vi "扫描脚本.vi"(4 "4-wire":bool, 6 "扫描":T1 {"测试参数"."反向极限电流(mA)" min=0.0 max=3000.0; "测试参数"."反向电压(V)" min=0.0 max=40.0; "测试参数"."正向极限电流(mA)" min=0.0 max=3000.0; "测试参数"."正向电压(V)" min=0.0 max=40.0; "时序参数"."反改变量(V)" min=0.0 max=40.0 step=5e-06; "时序参数"."正改变量(V)" min=0.0 max=40.0 step=5e-06; "时序参数"."nplc" min=0.001}, 8 "错误输入（无错误）":errorcluster, 11 "方向(T:正向)":bool=TRUE) -> (0 "错误输出":errorcluster, 1 "Script":string)   [LabVIEW 2021]
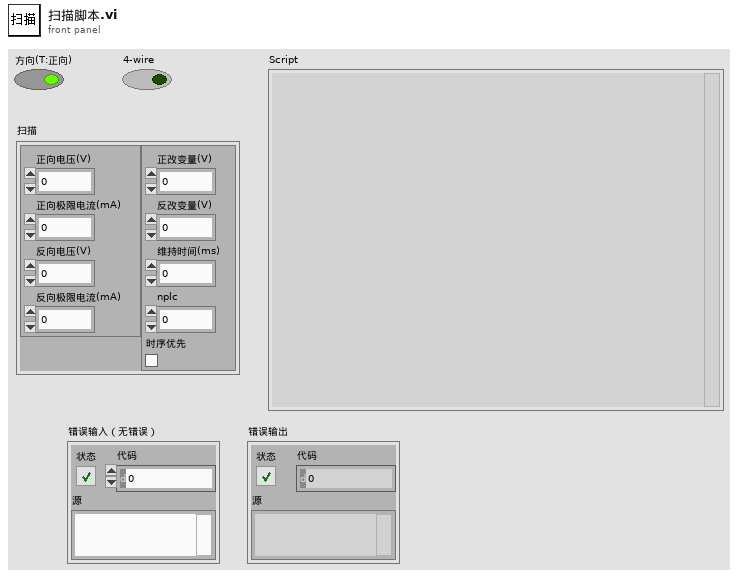
[diagram p1: front panel]
types:
  T1 = typedef "扫描参数.ctl" = cluster{"测试参数":cluster{"正向电压(V)":dbl, "正向极限电流(mA)":dbl, "反向电压(V)":dbl, "反向极限电流(mA)":dbl}, "时序参数":cluster{"正改变量(V)":dbl, "反改变量(V)":dbl, "维持时间(ms)":dbl, "nplc":dbl, "时序优先":bool}}
  T2 = cluster{"正改变量(V)":dbl, "反改变量(V)":dbl, "维持时间(ms)":dbl, "nplc":dbl, "时序优先":bool}
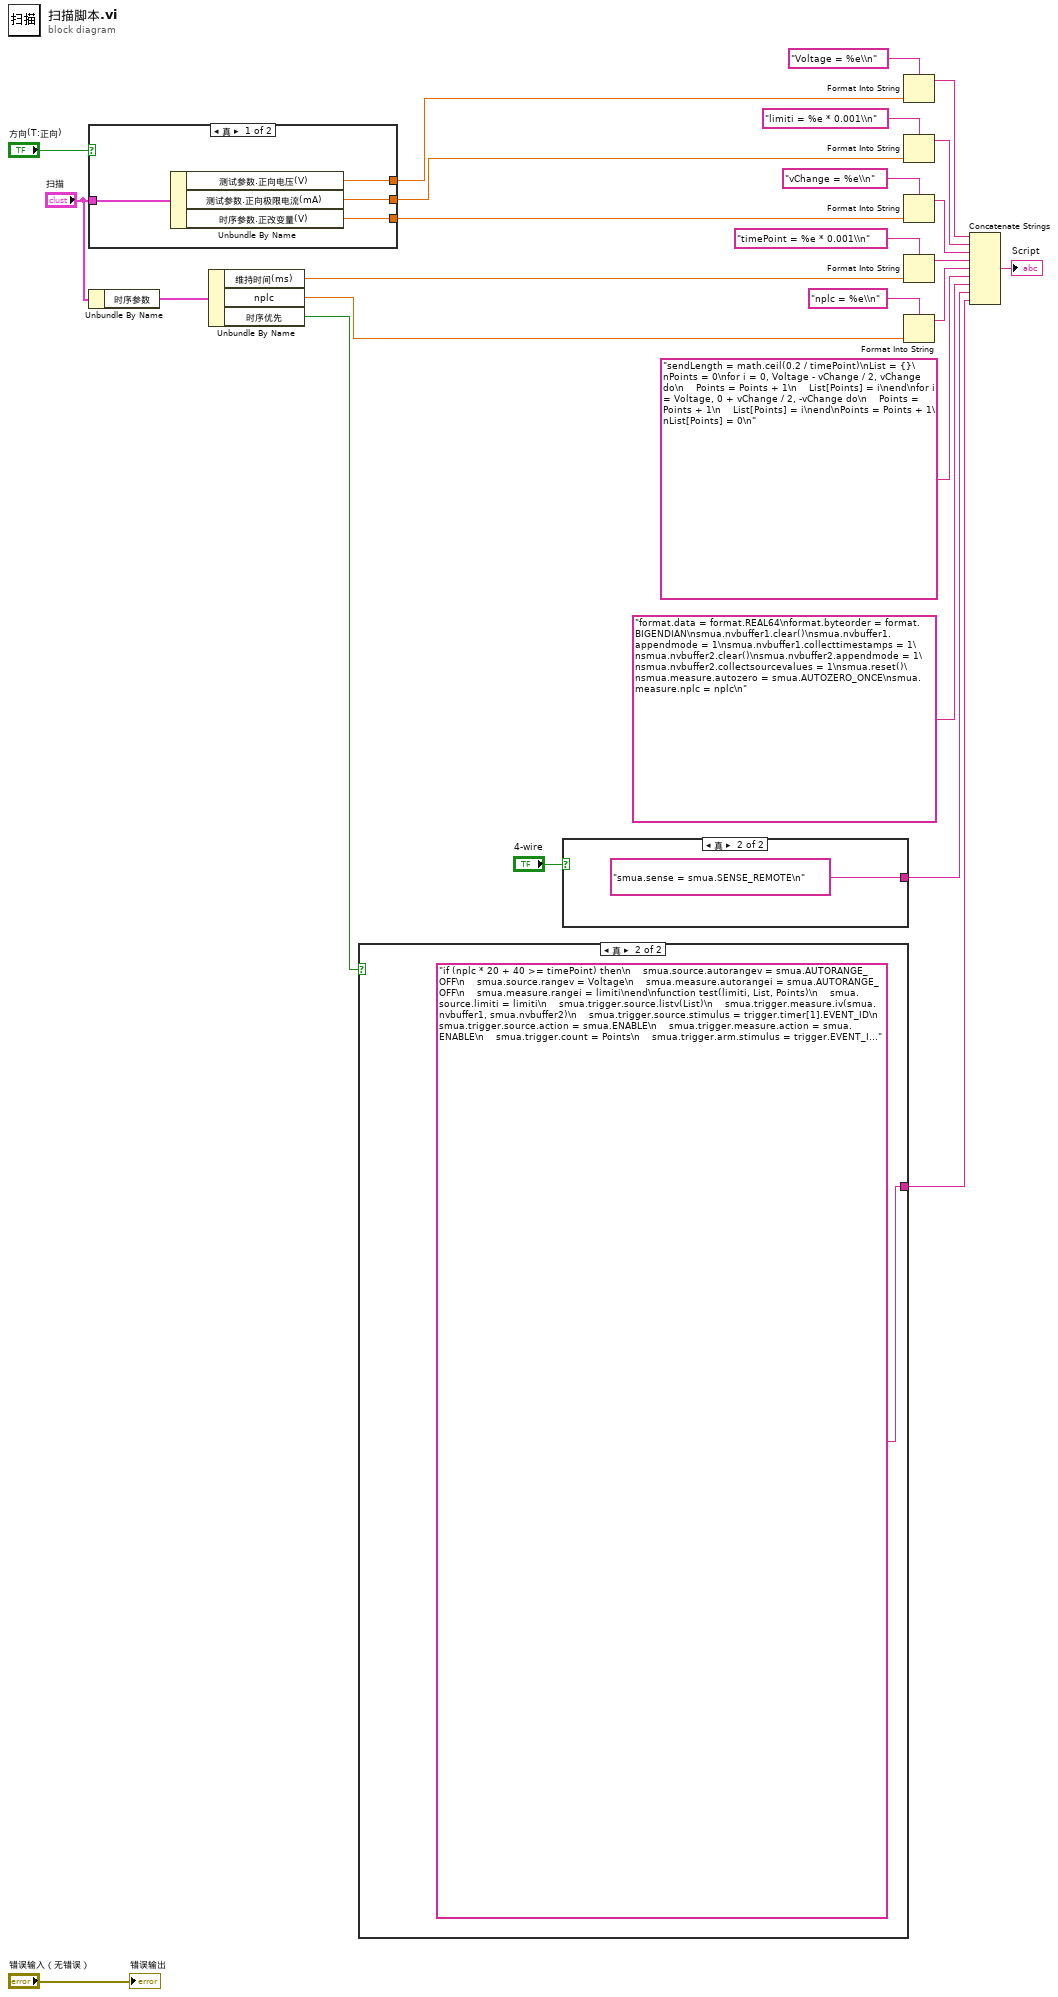
[diagram p0: block diagram]
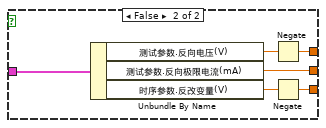
[diagram p2: hidden frame]
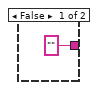
[diagram p3: hidden frame]
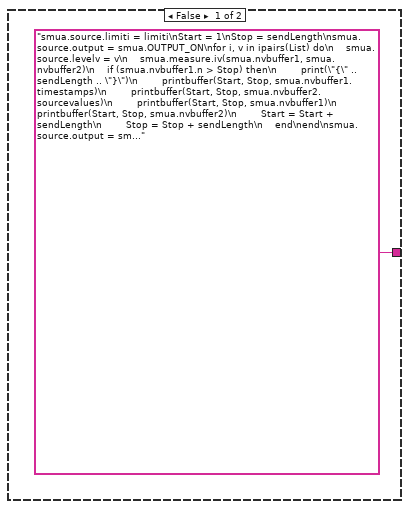
[diagram p4: hidden frame]
diagram:
  n1 = case shown="真" "方向(T:正向)" {
    tunnel: [w30 w35] -> w12
    tunnel: [w29 w32] -> w9
    tunnel: [w28 w33] -> w3
    tunnel: "扫描" -> [w27 w31]
    frame True {
      n2 = Unbundle By Name(w27) -> ("测试参数.正向电压(V)"=w30:dbl, "测试参数.正向极限电流(mA)"=w29:dbl, "时序参数.正改变量(V)"=w28:dbl)
    }
    frame False {
      n3 = Unbundle By Name(w31) -> ("测试参数.反向电压(V)"=w36:dbl, "测试参数.反向极限电流(mA)"=w32:dbl, "时序参数.反改变量(V)"=w34:dbl)
      n4 = Negate(x=w36) -> (-x=w35:dbl)
      n5 = Negate(x=w34) -> (-x=w33:dbl)
    }
  }
  n6 = Unbundle By Name("扫描") -> ("时序参数"=w15:T2)
  n7 = Unbundle By Name(w15) -> ("维持时间(ms)"=w5:dbl, "nplc"=w8:dbl, "时序优先"=w4:bool)
  n8 = case shown="真" w4 {
    tunnel: ["smua.source.limiti = limiti\nStart = 1\nStop = sendLength\nsmua.source.output = smua.OUTPUT_ON\nfor i, v in ipairs(List) do\n    smua.source.levelv = v\n    smua.measure.iv(smua.nvbuffer1, smua.nvbuffer2)\n    if (smua.nvbuffer1.n > Stop) then\n        print(\"{\" .. sendLength .. \"}\")\n        printbuffer(Start, Stop, smua.nvbuffer1.timestamps)\n        printbuffer(Start, Stop, smua.nvbuffer2.sourcevalues)\n        printbuffer(Start, Stop, smua.nvbuffer1)\n        printbuffer(Start, Stop, smua.nvbuffer2)\n        Start = Start + sendLength\n        Stop = Stop + sendLength\n    end\nend\nsmua.source.output = smua.OUTPUT_OFF\nStop = Points\nprint(\"{\" .. Stop - Start + 1 .. \"}\")\nprintbuffer(Start, Stop, smua.nvbuffer1.timestamps)\nprintbuffer(Start, Stop, smua.nvbuffer2.sourcevalues)\nprintbuffer(Start, Stop, smua.nvbuffer1)\nprintbuffer(Start, Stop, smua.nvbuffer2)\nprint(\"{done}\")\nreset()" "if (nplc * 20 + 40 >= timePoint) then\n    smua.source.autorangev = smua.AUTORANGE_OFF\n    smua.source.rangev = Voltage\n    smua.measure.autorangei = smua.AUTORANGE_OFF\n    smua.measure.rangei = limiti\nend\nfunction test(limiti, List, Points)\n    smua.source.limiti = limiti\n    smua.trigger.source.listv(List)\n    smua.trigger.measure.iv(smua.nvbuffer1, smua.nvbuffer2)\n    smua.trigger.source.stimulus = trigger.timer[1].EVENT_ID\n    smua.trigger.source.action = smua.ENABLE\n    smua.trigger.measure.action = smua.ENABLE\n    smua.trigger.count = Points\n    smua.trigger.arm.stimulus = trigger.EVENT_ID\n    trigger.timer[1].reset()\n    trigger.timer[1].stimulus = smua.trigger.ARMED_EVENT_ID\n    trigger.timer[1].passthrough = false\n    trigger.timer[1].delay = timePoint\n    trigger.timer[1].count = Points\n    smua.trigger.initiate()\n    smua.trigger.arm.set()\nend\nfunction sendData()\n    repeat\n        if (bit.test(status.operation.instrument.smua.condition, 4) == false) then\n            return\n        elseif (smua.nvbuffer1.n > Stop) then\n            print(\"{\" .. sendLength .. \"}\")\n            printbuffer(Start, Stop, smua.nvbuffer1.timestamps)\n            printbuffer(Start, Stop, smua.nvbuffer2.sourcevalues)\n            printbuffer(Start, Stop, smua.nvbuffer1)\n            printbuffer(Start, Stop, smua.nvbuffer2)\n            Start = Start + sendLength\n            Stop = Stop + sendLength\n        end\n        delay(timePoint)\n    until (false)\nend\nfunction sendLastData()\n    Stop = smua.nvbuffer1.n\n    print(\"{\" .. Stop - Start + 1 .. \"}\")\n    printbuffer(Start, Stop, smua.nvbuffer1.timestamps)\n    printbuffer(Start, Stop, smua.nvbuffer2.sourcevalues)\n    printbuffer(Start, Stop, smua.nvbuffer1)\n    printbuffer(Start, Stop, smua.nvbuffer2)\n    print(\"{done}\")\nend\nStart = 1\nStop = sendLength\nsmua.source.output = smua.OUTPUT_ON\ntest(limiti, List, Points)\nsendData()\nsmua.source.output = smua.OUTPUT_OFF\nsendLastData()\nreset()"] -> w18
    frame False {
    }
    frame True {
    }
  }
  n9 = case shown="真" "4-wire" {
    tunnel: ["" "smua.sense = smua.SENSE_REMOTE\n"] -> w17
    frame False {
    }
    frame True {
    }
  }
  n10 = Format Into String(format string="Voltage = %e\\n" ("格式字符串"), w12) -> (resulting string=w23:string)  [unwired: 2 in, 1 out]
  n11 = Format Into String(format string="limiti = %e * 0.001\\n" ("格式字符串"), w9) -> (resulting string=w10:string)  [unwired: 2 in, 1 out]
  n12 = Format Into String(format string="vChange = %e\\n" ("格式字符串"), w3) -> (resulting string=w11:string)  [unwired: 2 in, 1 out]
  n13 = Format Into String(format string="timePoint = %e * 0.001\\n", w5) -> (resulting string=w7:string)  [unwired: 2 in, 1 out]
  n14 = Format Into String(format string="nplc = %e\\n", w8) -> (resulting string=w6:string)  [unwired: 2 in, 1 out]
  n15 = Concatenate Strings(w23, w10, w11, w7, w6, "sendLength = math.ceil(0.2 / timePoint)\nList = {}\nPoints = 0\nfor i = 0, Voltage - vChange / 2, vChange do\n    Points = Points + 1\n    List[Points] = i\nend\nfor i = Voltage, 0 + vChange / 2, -vChange do\n    Points = Points + 1\n    List[Points] = i\nend\nPoints = Points + 1\nList[Points] = 0\n", "format.data = format.REAL64\nformat.byteorder = format.BIGENDIAN\nsmua.nvbuffer1.clear()\nsmua.nvbuffer1.appendmode = 1\nsmua.nvbuffer1.collecttimestamps = 1\nsmua.nvbuffer2.clear()\nsmua.nvbuffer2.appendmode = 1\nsmua.nvbuffer2.collectsourcevalues = 1\nsmua.reset()\nsmua.measure.autozero = smua.AUTOZERO_ONCE\nsmua.measure.nplc = nplc\n", w17, w18) -> (→"Script":string)
  "错误输出" <- "错误输入（无错误）"
